vi "Find Unique Properties in Category.vi"(10 "Unique Identifier":string, 11 "Front Panel Objects":refnum<vi>[](array[refnum])) -> (3 "Unique Properties in Category":string[](array[string]))   [LabVIEW 2019, in "LSS.lvlib"]
doc: "Finds a list of unique properties that apply to the front panel objects and share the unique identifier in their list of selectors.\n\n<b>Inputs:</b>\n<b>Front Panel Objects</b> - List of all front panel objects.\n<b>Unique Identifier</b> - Identifier to find within each objects list of selectors.\n\n<b>Outputs:</b>\n<b>Unique Properties in Category</b> - List of properties that apply to the front panel objects that share the unique identifier input."
uses:
  LSS.lvlib
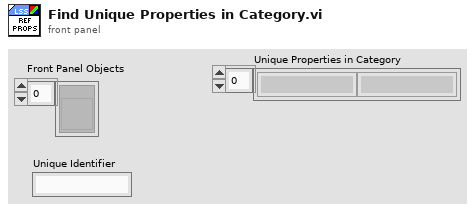
[diagram p1: front panel]
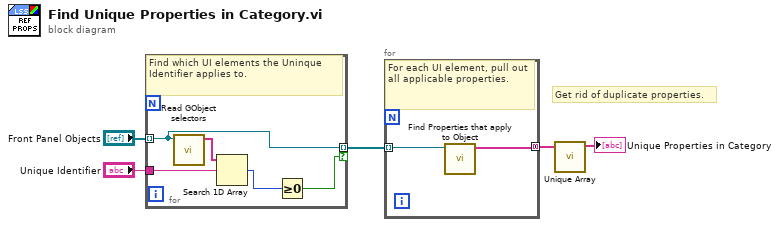
[diagram p0: block diagram]
diagram:
  # "Get rid of duplicate properties."
  n1 = for {
    tunnel: "Front Panel Objects" -> [w6] mode=indexing
    tunnel: [w6] -> w3 mode=indexing if=w7
    tunnel: "Unique Identifier" -> [w9]
    # "Find which UI elements the Uninque Identifier applies to."
    n2 = call "Read GObject selectors.vi"("Generic In"=w6) -> ("Selectors"=w10:string[])  [unwired: 9 in, 1 out]
    n3 = Search 1D Array(1D array=w10, element=w9) -> (index of element=w8:i32)  [unwired: 1 in]
    n4 = Greater Or Equal To 0?(x=w8) -> (x >= 0?=w7:bool)
  }
  n5 = for {
    tunnel: w3 -> [w12] mode=indexing
    tunnel: [w11] -> w2 mode=concatenating
    # "For each UI element, pull out all applicable properties."
    n6 = call "Find Properties that apply to Object.vi"("GObject in"=w12) -> ("Relevant Properties"=w11:string[])  [unwired: 10 in]
  }
  n7 = call "Unique Array.vi"("Array"=w2) -> ("Unique Array"=→"Unique Properties in Category":string[])  [unwired: 10 in]
